vi "tm3samp_framerate.vi"() -> ()   [LabVIEW 2011]
panel:
  out "Image":u16[][](graph)
  out "Camera Serial":string
  out "Camera Version":string
  out "Camera Model":string
  out "SMD":dbl
  in  "Scan Mode":dbl min=0.0 max=2.0 step=1.0
  in  "Exposure":dbl min=0.0010036691729323308 max=10.0 step=1e-08
  out "EXP":dbl
  out "SVW":i32
  out "SHW":i32
  out "SVO":i32
  out "SHO":i32
  in  "V Width":i32 min=4 max=2048 step=4
  in  "V Offset":i32 min=0 max=0 step=4
  in  "H Width":i32 min=4 max=2048 step=4
  in  "H Offset":i32 min=0 max=0 step=4
  in  "Binning":u16(ring) items=["1x1"=1, "2x2"=2, "4x4"=4]
  out "Elapsed Time":u32
  out "Total Frames":i32
  in  "Display":bool=TRUE
  out "Frames Per Second":dbl
  out "error out":errorcluster
  in  "stop":bool
  # "This example displays the frame rate\nof the camera.  Changing the resolution\nof the camera or displaying the images\nwill affect the frame rate."
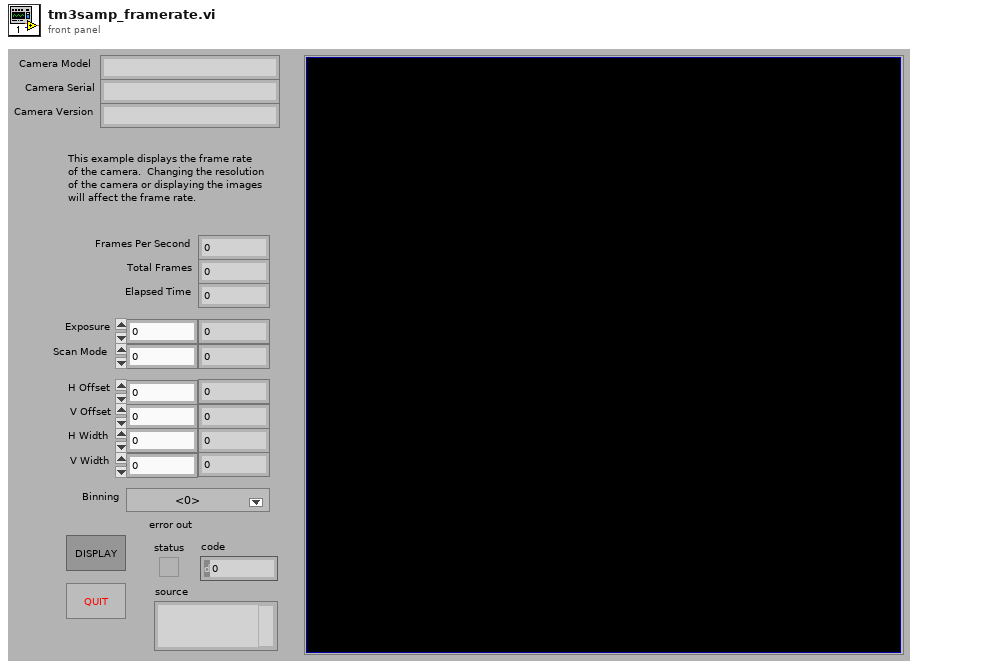
[diagram p1: front panel]
types:
  T1 = cluster{"Value":i32, "Minimum":i32, "Maximum":i32, "Increment":i32}
  T2 = cluster{"width":u32, "height":u32, "datatype":u32}
  T3 = cluster{"H Offset":i32, "V Offset":i32, "H Width":i32, "V Width":i32}
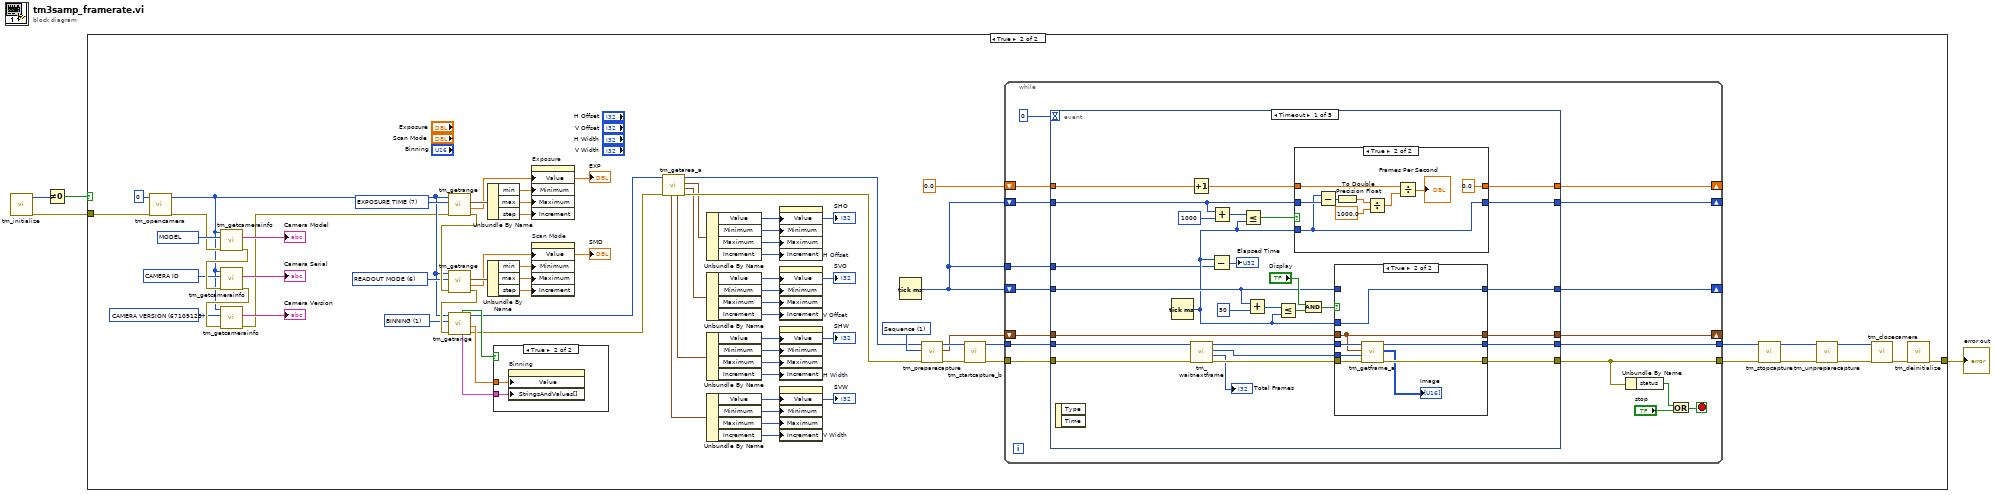
[diagram p0: block diagram]
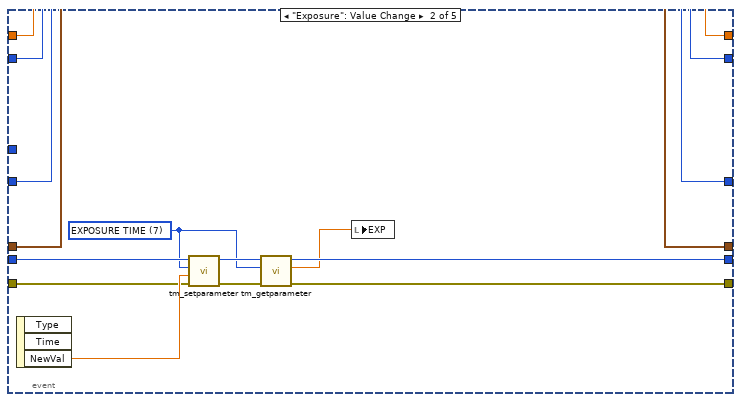
[diagram p6: hidden frame]
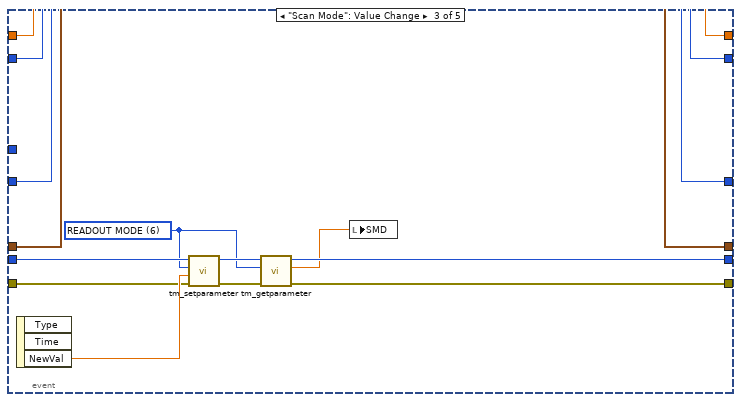
[diagram p7: hidden frame]
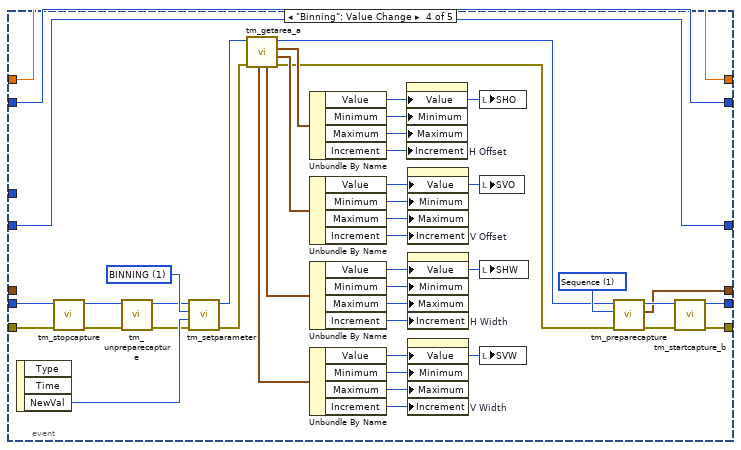
[diagram p8: hidden frame]
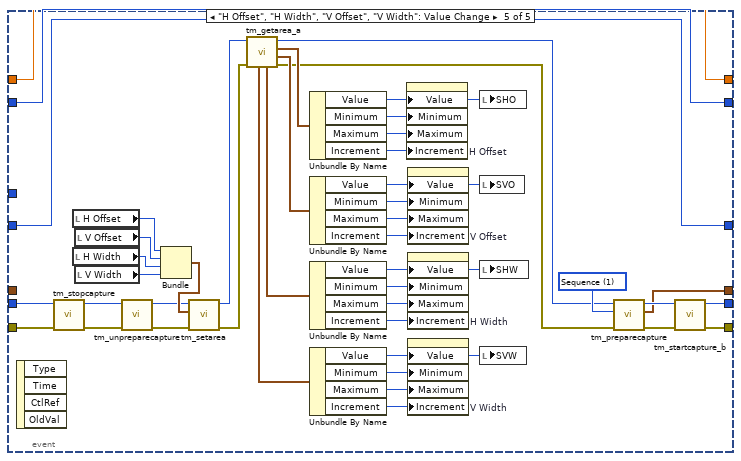
[diagram p9: hidden frame]
diagram:
  n1 = call <userlib>:"tm_initialize.vi"() -> ("error out"=w2:errorcluster, "Number Of Cameras"=w1:u32)  [unwired: 10 in]
  n2 = Not Equal To 0?(x=w1) -> (x != 0?=w4:bool)
  n3 = case shown="True" w4 {
    tunnel: [w5 w73] -> w3
    tunnel: w2 -> [w5 w76]
    frame False {
    }
    frame True {
      w19 = u32 67109122 items=["BUS"=67109121, "CAMERA ID"=67109122, "VENDOR"=67109123, "MODEL"=67109124, "CAMERA VERSION"=67109125, "DRIVER VERSION"=67109126, "MODULE VERSIOIN"=67109127, "DCAMAPI VERSION"=67109128] ("Info ID")
      w24 = u32 67109125 items=["BUS"=67109121, "CAMERA"=67109122, "VENDOR"=67109123, "MODEL"=67109124, "CAMERA VERSION"=67109125, "DRIVER VERSION"=67109126, "MODULE VERSIOIN"=67109127, "DCAMAPI VERSION"=67109128] ("Info ID")
      w27 = u32 67109124 items=["BUS"=67109121, "CAMERA"=67109122, "VENDOR"=67109123, "MODEL"=67109124, "CAMERA VERSION"=67109125, "DRIVER VERSION"=67109126, "MODULE VERSIOIN"=67109127, "DCAMAPI VERSION"=67109128] ("Info ID")
      w59 = 1 items=["BINNING"=1, "BITS PER CHANNEL"=2, "ACTIVE VIEW INDEX"=3, "CCD MODE"=4, "SENSOR MODE"=5, "READOUT MODE"=6, "EXPOSURE TIME"=7, "CONTRAST GAIN"=8, "CONTRAST OFFSET"=9, "LIGHT MODE"=10, "SENSITIVITY"=11, "WHITE BALANCE"=12, "PHOTON IMAGING MODE"=13, "HIGH DYNAMIC RANGE MODE"=14, "TRIGGER SOURCE"=15, "TRIGGER ACTIVE"=16, "TRIGGER MODE"=17, "TRIGGER POLARITY"=18, "TRIGGER GLOBAL EXPOSURE"=19, "FIRST TRIGGER BEHAVIOR"=20, "TRIGGER TIMES"=21, "OUTPUT TRIGGER POLARITY"=22, "OUTPUT TRIGGER DELAY"=23, "OUTPUT TRIGGER PERIOD"=24, "TEMPERATURE"=25, "TEMPERATURE TARGET"=26, "SENSOR COOLER FAN"=27, "MECHANICAL SHUTTER"=28, "BACK FOCUS POSITION"=29, "FRAMEBUNDLE MODE"=30, "FRAMEBUNDLE NUMBER"=31] ("Parameter")
      w61 = 6 items=["BINNING"=1, "BITS PER CHANNEL"=2, "ACTIVE VIEW INDEX"=3, "CCD MODE"=4, "SENSOR MODE"=5, "READOUT MODE"=6, "EXPOSURE TIME"=7, "CONTRAST GAIN"=8, "CONTRAST OFFSET"=9, "LIGHT MODE"=10, "SENSITIVITY"=11, "WHITE BALANCE"=12, "PHOTON IMAGING MODE"=13, "HIGH DYNAMIC RANGE MODE"=14, "TRIGGER SOURCE"=15, "TRIGGER ACTIVE"=16, "TRIGGER MODE"=17, "TRIGGER POLARITY"=18, "TRIGGER GLOBAL EXPOSURE"=19, "FIRST TRIGGER BEHAVIOR"=20, "TRIGGER TIMES"=21, "OUTPUT TRIGGER POLARITY"=22, "OUTPUT TRIGGER DELAY"=23, "OUTPUT TRIGGER PERIOD"=24, "TEMPERATURE"=25, "TEMPERATURE TARGET"=26, "SENSOR COOLER FAN"=27, "MECHANICAL SHUTTER"=28, "BACK FOCUS POSITION"=29, "FRAMEBUNDLE MODE"=30, "FRAMEBUNDLE NUMBER"=31] ("Parameter")
      w64 = 7 items=["BINNING"=1, "BITS PER CHANNEL"=2, "ACTIVE VIEW INDEX"=3, "CCD MODE"=4, "SENSOR MODE"=5, "READOUT MODE"=6, "EXPOSURE TIME"=7, "CONTRAST GAIN"=8, "CONTRAST OFFSET"=9, "LIGHT MODE"=10, "SENSITIVITY"=11, "WHITE BALANCE"=12, "PHOTON IMAGING MODE"=13, "HIGH DYNAMIC RANGE MODE"=14, "TRIGGER SOURCE"=15, "TRIGGER ACTIVE"=16, "TRIGGER MODE"=17, "TRIGGER POLARITY"=18, "TRIGGER GLOBAL EXPOSURE"=19, "FIRST TRIGGER BEHAVIOR"=20, "TRIGGER TIMES"=21, "OUTPUT TRIGGER POLARITY"=22, "OUTPUT TRIGGER DELAY"=23, "OUTPUT TRIGGER PERIOD"=24, "TEMPERATURE"=25, "TEMPERATURE TARGET"=26, "SENSOR COOLER FAN"=27, "MECHANICAL SHUTTER"=28, "BACK FOCUS POSITION"=29, "FRAMEBUNDLE MODE"=30, "FRAMEBUNDLE NUMBER"=31] ("Parameter")
      w71 = 1 items=["Snap", "Sequence"] ("Capture mode")
      n4 = call <userlib>:"tm_opencamera.vi"("error in (no error)"=w76, "Camera Index"=u32 0) -> ("error out"=w20:errorcluster, "Handle out"=w7:u32)  [unwired: 8 in]
      n5 = call <userlib>:"tm_getcamerainfo.vi"("error in (no error)"=w20, "Info ID"=w27, "Handle in"=w7) -> ("error out"=w26:errorcluster, "String"=→"Camera Model":string)  [unwired: 6 in, 1 out]
      n6 = call <userlib>:"tm_getcamerainfo.vi"("error in (no error)"=w26, "Info ID"=w19, "Handle in"=w7) -> ("error out"=w25:errorcluster, "String"=→"Camera Serial":string)  [unwired: 6 in, 1 out]
      n7 = call <userlib>:"tm_getcamerainfo.vi"("error in (no error)"=w25, "Info ID"=w24, "Handle in"=w7) -> ("error out"=w6:errorcluster, "String"=→"Camera Version":string)  [unwired: 6 in, 1 out]
      n8 = call <userlib>:"tm_getrange.vi"("error in (no error)"=w6, "Parameter"=w64, "Handle in"=w7) -> ("error out"=w62:errorcluster, "default"=w55:dbl, "Range"=w63:cluster{"min":dbl, "max":dbl, "step":dbl})  [unwired: 2 in, 4 out]
      "EXP" <- w55
      n9 = call <userlib>:"tm_getrange.vi"("error in (no error)"=w62, "Parameter"=w61, "Handle in"=w7) -> ("error out"=w60:errorcluster, "default"=w50:dbl, "Range"=w54:cluster{"min":dbl, "max":dbl, "step":dbl})  [unwired: 2 in, 4 out]
      "SMD" <- w50
      n10 = call <userlib>:"tm_getrange.vi"("error in (no error)"=w60, "Parameter"=w59, "Handle in"=w7) -> ("error out"=w45:errorcluster, "default"=w47:dbl, "Handle out"=w46:u32, "Value Names"=w48:cluster{"Name":string, "Value":dbl}[], "Writable"=w49:bool)  [unwired: 2 in, 2 out]
      n11 = Unbundle By Name(w63) -> ("min"=w58:dbl, "max"=w57:dbl, "step"=w56:dbl)
      n12 = Unbundle By Name(w54) -> ("min"=w53:dbl, "max"=w52:dbl, "step"=w51:dbl)
      n13 = case shown="True" w49 {
        tunnel: w48 -> [_ w78]
        tunnel: w47 -> [_ w77]
        frame False {
        }
        frame True {
          n14 = property on="Binning" class="Ring (strict)"("Value"=w77, "StringsAndValues[]"=w78) -> ()  [unwired: 2 in, 2 out]
        }
      }
      n15 = property on="Exposure" class="DigNum (strict)"("Value"=w55, "Minimum"=w58, "Maximum"=w57, "Increment"=w56) -> ()  [unwired: 2 in, 2 out]
      n16 = property on="Scan Mode" class="DigNum (strict)"("Value"=w50, "Minimum"=w53, "Maximum"=w52, "Increment"=w51) -> ()  [unwired: 2 in, 2 out]
      n17 = call <userlib>:"tm_getarea_a.vi"("error in (no error)"=w45, "Handle in"=w46) -> ("error out"=w43:errorcluster, "V Offset"=w42:T1, "H Offset"=w12:T1, "Handle out"=w44:u32, "H Width"=w41:T1, "V Width"=w40:T1)  [unwired: 4 in]
      n18 = Unbundle By Name(w12) -> ("Value"=w11:i32, "Minimum"=w10:i32, "Maximum"=w9:i32, "Increment"=w8:i32)
      "SHO" <- w11
      n19 = Unbundle By Name(w42) -> ("Value"=w30:i32, "Minimum"=w39:i32, "Maximum"=w38:i32, "Increment"=w37:i32)
      "SVO" <- w30
      n20 = Unbundle By Name(w41) -> ("Value"=w29:i32, "Minimum"=w36:i32, "Maximum"=w35:i32, "Increment"=w34:i32)
      "SHW" <- w29
      n21 = Unbundle By Name(w40) -> ("Value"=w28:i32, "Minimum"=w33:i32, "Maximum"=w32:i32, "Increment"=w31:i32)
      "SVW" <- w28
      n22 = property on="H Offset" class="DigNum (strict)"("Value"=w11, "Minimum"=w10, "Maximum"=w9, "Increment"=w8) -> ()  [unwired: 2 in, 2 out]
      n23 = property on="V Offset" class="DigNum (strict)"("Value"=w30, "Minimum"=w39, "Maximum"=w38, "Increment"=w37) -> ()  [unwired: 2 in, 2 out]
      n24 = property on="H Width" class="DigNum (strict)"("Value"=w29, "Minimum"=w36, "Maximum"=w35, "Increment"=w34) -> ()  [unwired: 2 in, 2 out]
      n25 = property on="V Width" class="DigNum (strict)"("Value"=w28, "Minimum"=w33, "Maximum"=w32, "Increment"=w31) -> ()  [unwired: 2 in, 2 out]
      n26 = Tick Count (ms)() -> (millisecond timer value=w65:u32)
      n27 = call <userlib>:"tm_preparecapture.vi"("error in (no error)"=w43, "Capture mode"=w71, "Handle in"=w44) -> ("error out"=w69:errorcluster, "Buffer"=w66:T2, "Handle out"=w70:u32)  [unwired: 5 in, 1 out]
      n28 = call <userlib>:"tm_startcapture_b.vi"("error in (no error)"=w69, "Handle in"=w70) -> ("error out"=w68:errorcluster, "Handle out"=w67:u32)  [unwired: 8 in]
      n29 = while {
        tunnel: w68 -> [w83]
        tunnel: [w81] -> w18
        tunnel: [w80] -> w17
        shift-right: [w90] -> _
        shift-left: w65 -> [w88]
        shift-right: [w91] -> _
        shift-left: 0.0 -> [w89]
        shift-right: [w82] -> _
        shift-left: w65 -> [w86]
        tunnel: w67 -> [w84]
        tunnel: w65 -> [w87]
        shift-right: [w79] -> _
        shift-left: w66 -> [w85]
        stop <- w93 stop-if-true
        n30 = event shown="[0] Timeout" {
          selector: _ -> [_ _ _ _ _]
          dyn-events: _ -> [_ _ _ _ _]
          timeout: 0 -> [_ _ _ _ _]
          tunnel: [w103 w156 w169 w203 w249] -> w91
          tunnel: [w102 w157 w170 w204 w250] -> w90
          tunnel: w89 -> [w104 w156 w169 w203 w249]
          tunnel: w88 -> [w106 w157 w170 w204 w250]
          tunnel: w87 -> [w98 _ _ _ _]
          tunnel: w86 -> [w107 w159 w172 w213 w257]
          tunnel: w85 -> [w97 w148 w161 _ _]
          tunnel: w84 -> [w109 w154 w167 w178 w219]
          tunnel: w83 -> [w108 w155 w168 w177 w218]
          tunnel: [w101 w159 w172 w213 w257] -> w82
          tunnel: [w100 w150 w163 w207 w252] -> w81
          tunnel: [w99 w149 w162 w208 w253] -> w80
          tunnel: [w96 w148 w161 w206 w251] -> w79
          event Timeout {
            n31 = event-data() -> ()  [unwired: 1 in, 2 out]
            n32 = Tick Count (ms)() -> (millisecond timer value=w105:u32)
            n33 = Increment(x=w104) -> (x+1=w120:dbl)
            n34 = call <userlib>:"tm_waitnextframe.vi"("error in (no error)"=w108, "Handle in"=w109) -> ("error out"=w114:errorcluster, "Frame Count"=→"Total Frames":i32, "Frame Index"=w113:i32, "Handle out"=w115:u32)  [unwired: 6 in]
            n35 = Subtract(x=w105, y=w98) -> (x-y=→"Elapsed Time":u32)
            n36 = Add(x=w106, y=u32 1000) -> (x+y=w123:u32)
            n37 = Less Or Equal?(x=w123, y=w105) -> (x <= y?=w122:bool)
            n38 = Add(x=w107, y=u32 50) -> (x+y=w119:u32)
            n39 = Less Or Equal?(x=w119, y=w105) -> (x <= y?=w117:bool)
            n40 = case shown="True" w122 {
              tunnel: w106 -> [w137 w140]
              tunnel: [w137 w138] -> w102
              tunnel: w120 -> [w136 w144]
              tunnel: w105 -> [_ w138]
              tunnel: [w136 0.0] -> w103
              frame False {
              }
              frame True {
                n41 = Subtract(x=w138, y=w140) -> (x-y=w139:u32)
                n42 = To Double Precision Float(number=w139) -> (double precision float=w146:dbl)
                n43 = Divide(x=w146, y=1000.0) -> (x/y=w143:dbl)
                n44 = Divide(x=w144, y=w143) -> (x/y=→"Frames Per Second":dbl)
              }
            }
            n45 = And(x="Display", y=w117) -> (x .and. y?=w112:bool)
            n46 = case shown="True" w112 {
              tunnel: w107 -> [w127 _]
              tunnel: w105 -> [_ w135]
              tunnel: [w127 w135] -> w101
              tunnel: w115 -> [w126 w134]
              tunnel: w97 -> [w124 w129]
              tunnel: w114 -> [w125 w133]
              tunnel: [w126 w132] -> w100
              tunnel: [w125 w131] -> w99
              tunnel: w113 -> [_ w130]
              tunnel: [w124 w129] -> w96
              frame False {
              }
              frame True {
                n47 = call <userlib>:"tm_getframe_a.vi"("error in (no error)"=w133, "Frame Index"=w130, "Buffer"=w129, "Handle in"=w134) -> ("error out"=w131:errorcluster, "Data 16"=→"Image":u16[][], "Handle out"=w132:u32)  [unwired: 3 in, 2 out]
              }
            }
          }
          event "Exposure": Value Change {
            w151 = 7 items=["BINNING"=1, "BITS PER CHANNEL"=2, "ACTIVE VIEW INDEX"=3, "CCD MODE"=4, "SENSOR MODE"=5, "READOUT MODE"=6, "EXPOSURE TIME"=7, "CONTRAST GAIN"=8, "CONTRAST OFFSET"=9, "LIGHT MODE"=10, "SENSITIVITY"=11, "WHITE BALANCE"=12, "PHOTON IMAGING MODE"=13, "HIGH DYNAMIC RANGE MODE"=14, "TRIGGER SOURCE"=15, "TRIGGER ACTIVE"=16, "TRIGGER MODE"=17, "TRIGGER POLARITY"=18, "TRIGGER GLOBAL EXPOSURE"=19, "FIRST TRIGGER BEHAVIOR"=20, "TRIGGER TIMES"=21, "OUTPUT TRIGGER POLARITY"=22, "OUTPUT TRIGGER DELAY"=23, "OUTPUT TRIGGER PERIOD"=24, "TEMPERATURE"=25, "TEMPERATURE TARGET"=26, "SENSOR COOLER FAN"=27, "MECHANICAL SHUTTER"=28, "BACK FOCUS POSITION"=29, "FRAMEBUNDLE MODE"=30, "FRAMEBUNDLE NUMBER"=31] ("Parameter")
            n48 = event-data() -> ("NewVal"=w158:dbl)  [unwired: 1 in, 2 out]
            n49 = call <userlib>:"tm_setparameter.vi"("error in (no error)"=w155, "Value in"=w158, "Parameter"=w151, "Handle in"=w154) -> ("error out"=w153:errorcluster, "Handle out"=w152:u32)  [unwired: 6 in]
            n50 = call <userlib>:"tm_getparameter.vi"("error in (no error)"=w153, "Parameter"=w151, "Handle in"=w152) -> ("error out"=w149:errorcluster, "Value out"=w147:dbl, "Handle out"=w150:u32)  [unwired: 6 in]
            n51 = local write "EXP"(w147) -> ()
          }
          event "Scan Mode": Value Change {
            w164 = 6 items=["BINNING"=1, "BITS PER CHANNEL"=2, "ACTIVE VIEW INDEX"=3, "CCD MODE"=4, "SENSOR MODE"=5, "READOUT MODE"=6, "EXPOSURE TIME"=7, "CONTRAST GAIN"=8, "CONTRAST OFFSET"=9, "LIGHT MODE"=10, "SENSITIVITY"=11, "WHITE BALANCE"=12, "PHOTON IMAGING MODE"=13, "HIGH DYNAMIC RANGE MODE"=14, "TRIGGER SOURCE"=15, "TRIGGER ACTIVE"=16, "TRIGGER MODE"=17, "TRIGGER POLARITY"=18, "TRIGGER GLOBAL EXPOSURE"=19, "FIRST TRIGGER BEHAVIOR"=20, "TRIGGER TIMES"=21, "OUTPUT TRIGGER POLARITY"=22, "OUTPUT TRIGGER DELAY"=23, "OUTPUT TRIGGER PERIOD"=24, "TEMPERATURE"=25, "TEMPERATURE TARGET"=26, "SENSOR COOLER FAN"=27, "MECHANICAL SHUTTER"=28, "BACK FOCUS POSITION"=29, "FRAMEBUNDLE MODE"=30, "FRAMEBUNDLE NUMBER"=31] ("Parameter")
            n52 = event-data() -> ("NewVal"=w171:dbl)  [unwired: 1 in, 2 out]
            n53 = call <userlib>:"tm_setparameter.vi"("error in (no error)"=w168, "Value in"=w171, "Parameter"=w164, "Handle in"=w167) -> ("error out"=w166:errorcluster, "Handle out"=w165:u32)  [unwired: 6 in]
            n54 = call <userlib>:"tm_getparameter.vi"("error in (no error)"=w166, "Parameter"=w164, "Handle in"=w165) -> ("error out"=w162:errorcluster, "Value out"=w160:dbl, "Handle out"=w163:u32)  [unwired: 6 in]
            n55 = local write "SMD"(w160) -> ()
          }
          event "Binning": Value Change {
            w211 = 1 items=["Snap", "Sequence"] ("Capture mode")
            w212 = 1 items=["BINNING"=1, "BITS PER CHANNEL"=2, "ACTIVE VIEW INDEX"=3, "CCD MODE"=4, "SENSOR MODE"=5, "READOUT MODE"=6, "EXPOSURE TIME"=7, "CONTRAST GAIN"=8, "CONTRAST OFFSET"=9, "LIGHT MODE"=10, "SENSITIVITY"=11, "WHITE BALANCE"=12, "PHOTON IMAGING MODE"=13, "HIGH DYNAMIC RANGE MODE"=14, "TRIGGER SOURCE"=15, "TRIGGER ACTIVE"=16, "TRIGGER MODE"=17, "TRIGGER POLARITY"=18, "TRIGGER GLOBAL EXPOSURE"=19, "FIRST TRIGGER BEHAVIOR"=20, "TRIGGER TIMES"=21, "OUTPUT TRIGGER POLARITY"=22, "OUTPUT TRIGGER DELAY"=23, "OUTPUT TRIGGER PERIOD"=24, "TEMPERATURE"=25, "TEMPERATURE TARGET"=26, "SENSOR COOLER FAN"=27, "MECHANICAL SHUTTER"=28, "BACK FOCUS POSITION"=29, "FRAMEBUNDLE MODE"=30, "FRAMEBUNDLE NUMBER"=31] ("Parameter")
            n56 = event-data() -> ("NewVal"=w205:u16)  [unwired: 1 in, 2 out]
            n57 = call <userlib>:"tm_stopcapture.vi"("error in (no error)"=w177, "Handle in"=w178) -> ("error out"=w173:errorcluster, "Handle out"=w176:u32)  [unwired: 8 in]
            n58 = call <userlib>:"tm_unpreparecapture.vi"("error in (no error)"=w173, "Handle in"=w176) -> ("error out"=w174:errorcluster, "Handle out"=w175:u32)  [unwired: 8 in]
            n59 = call <userlib>:"tm_setparameter.vi"("error in (no error)"=w174, "Value in"=w205, "Parameter"=w212, "Handle in"=w175) -> ("error out"=w197:errorcluster, "Handle out"=w198:u32)  [unwired: 6 in]
            n60 = call <userlib>:"tm_getarea_a.vi"("error in (no error)"=w197, "Handle in"=w198) -> ("error out"=w196:errorcluster, "V Offset"=w200:T1, "H Offset"=w199:T1, "Handle out"=w195:u32, "H Width"=w201:T1, "V Width"=w202:T1)  [unwired: 4 in]
            n61 = Unbundle By Name(w199) -> ("Value"=w191:i32, "Minimum"=w194:i32, "Maximum"=w193:i32, "Increment"=w192:i32)
            n62 = Unbundle By Name(w200) -> ("Value"=w181:i32, "Minimum"=w190:i32, "Maximum"=w189:i32, "Increment"=w188:i32)
            n63 = Unbundle By Name(w201) -> ("Value"=w180:i32, "Minimum"=w187:i32, "Maximum"=w186:i32, "Increment"=w185:i32)
            n64 = Unbundle By Name(w202) -> ("Value"=w179:i32, "Minimum"=w184:i32, "Maximum"=w183:i32, "Increment"=w182:i32)
            n65 = property on="H Offset" class="DigNum (strict)"("Value"=w191, "Minimum"=w194, "Maximum"=w193, "Increment"=w192) -> ()  [unwired: 2 in, 2 out]
            n66 = property on="V Offset" class="DigNum (strict)"("Value"=w181, "Minimum"=w190, "Maximum"=w189, "Increment"=w188) -> ()  [unwired: 2 in, 2 out]
            n67 = property on="H Width" class="DigNum (strict)"("Value"=w180, "Minimum"=w187, "Maximum"=w186, "Increment"=w185) -> ()  [unwired: 2 in, 2 out]
            n68 = property on="V Width" class="DigNum (strict)"("Value"=w179, "Minimum"=w184, "Maximum"=w183, "Increment"=w182) -> ()  [unwired: 2 in, 2 out]
            n69 = local write "SHO"(w191) -> ()
            n70 = local write "SVO"(w181) -> ()
            n71 = local write "SHW"(w180) -> ()
            n72 = local write "SVW"(w179) -> ()
            n73 = call <userlib>:"tm_preparecapture.vi"("error in (no error)"=w196, "Capture mode"=w211, "Handle in"=w195) -> ("error out"=w209:errorcluster, "Buffer"=w206:T2, "Handle out"=w210:u32)  [unwired: 5 in, 1 out]
            n74 = call <userlib>:"tm_startcapture_b.vi"("error in (no error)"=w209, "Handle in"=w210) -> ("error out"=w208:errorcluster, "Handle out"=w207:u32)  [unwired: 8 in]
          }
          event "H Offset", "H Width", "V Offset", "V Width": Value Change {
            w256 = 1 items=["Snap", "Sequence"] ("Capture mode")
            n75 = event-data() -> ()  [unwired: 1 in, 4 out]
            n76 = call <userlib>:"tm_stopcapture.vi"("error in (no error)"=w218, "Handle in"=w219) -> ("error out"=w216:errorcluster, "Handle out"=w217:u32)  [unwired: 8 in]
            n77 = local read "H Offset"() -> (w222:i32)
            n78 = local read "H Width"() -> (w223:i32)
            n79 = local read "V Offset"() -> (w224:i32)
            n80 = local read "V Width"() -> (w221:i32)
            n81 = call <userlib>:"tm_unpreparecapture.vi"("error in (no error)"=w216, "Handle in"=w217) -> ("error out"=w214:errorcluster, "Handle out"=w215:u32)  [unwired: 8 in]
            n82 = Bundle("H Offset"=w222, "V Offset"=w224, "H Width"=w223, "V Width"=w221) -> (w220:T3)  [unwired: 1 in]
            n83 = call <userlib>:"tm_setarea.vi"("error in (no error)"=w214, "Sub Region"=w220, "Handle in"=w215) -> ("error out"=w225:errorcluster, "Handle out"=w226:u32)  [unwired: 7 in]
            n84 = call <userlib>:"tm_getarea_a.vi"("error in (no error)"=w225, "Handle in"=w226) -> ("error out"=w244:errorcluster, "V Offset"=w246:T1, "H Offset"=w245:T1, "Handle out"=w243:u32, "H Width"=w247:T1, "V Width"=w248:T1)  [unwired: 4 in]
            n85 = Unbundle By Name(w245) -> ("Value"=w239:i32, "Minimum"=w242:i32, "Maximum"=w241:i32, "Increment"=w240:i32)
            n86 = Unbundle By Name(w246) -> ("Value"=w229:i32, "Minimum"=w238:i32, "Maximum"=w237:i32, "Increment"=w236:i32)
            n87 = Unbundle By Name(w247) -> ("Value"=w228:i32, "Minimum"=w235:i32, "Maximum"=w234:i32, "Increment"=w233:i32)
            n88 = Unbundle By Name(w248) -> ("Value"=w227:i32, "Minimum"=w232:i32, "Maximum"=w231:i32, "Increment"=w230:i32)
            n89 = property on="H Offset" class="DigNum (strict)"("Value"=w239, "Minimum"=w242, "Maximum"=w241, "Increment"=w240) -> ()  [unwired: 2 in, 2 out]
            n90 = property on="V Offset" class="DigNum (strict)"("Value"=w229, "Minimum"=w238, "Maximum"=w237, "Increment"=w236) -> ()  [unwired: 2 in, 2 out]
            n91 = property on="H Width" class="DigNum (strict)"("Value"=w228, "Minimum"=w235, "Maximum"=w234, "Increment"=w233) -> ()  [unwired: 2 in, 2 out]
            n92 = property on="V Width" class="DigNum (strict)"("Value"=w227, "Minimum"=w232, "Maximum"=w231, "Increment"=w230) -> ()  [unwired: 2 in, 2 out]
            n93 = local write "SHO"(w239) -> ()
            n94 = local write "SVO"(w229) -> ()
            n95 = local write "SHW"(w228) -> ()
            n96 = local write "SVW"(w227) -> ()
            n97 = call <userlib>:"tm_preparecapture.vi"("error in (no error)"=w244, "Capture mode"=w256, "Handle in"=w243) -> ("error out"=w254:errorcluster, "Buffer"=w251:T2, "Handle out"=w255:u32)  [unwired: 5 in, 1 out]
            n98 = call <userlib>:"tm_startcapture_b.vi"("error in (no error)"=w254, "Handle in"=w255) -> ("error out"=w253:errorcluster, "Handle out"=w252:u32)  [unwired: 8 in]
          }
        }
        n99 = Unbundle By Name(w80) -> ("status"=w94:bool)
        n100 = Or(x=w94, y="stop") -> (x .or. y?=w93:bool)
      }
      n101 = call <userlib>:"tm_stopcapture.vi"("error in (no error)"=w17, "Handle in"=w18) -> ("error out"=w14:errorcluster, "Handle out"=w15:u32)  [unwired: 8 in]
      n102 = call <userlib>:"tm_unpreparecapture.vi"("error in (no error)"=w14, "Handle in"=w15) -> ("error out"=w13:errorcluster, "Handle out"=w16:u32)  [unwired: 8 in]
      n103 = call <userlib>:"tm_closecamera.vi"("error in (no error)"=w13, "Handle in"=w16) -> ("error out"=w74:errorcluster)  [unwired: 9 in]
      n104 = call <userlib>:"tm_deinitialize.vi"("error in (no error)"=w74) -> ("error out"=w73:errorcluster)  [unwired: 10 in]
    }
  }
  "error out" <- w3
